vi "wfm_feature update_xygraph_x_scale.vi"(8 "error in (no error)":errorcluster, 10 "NewRange":T1, 11 "wfm_feature in":refnum<class "wfm_feature.lvclass">) -> (0 "error out":errorcluster, 3 "wfm_feature out":refnum<class "wfm_feature.lvclass">)   [LabVIEW 2018, in "wfm_feature.lvclass"]
uses:
  wfm_feature.lvclass
  <vilib>/Utility/miscctls.llb/LVRangeTypeDef.ctl
  wfm_feature.lvclass/wfm_feature.ctl
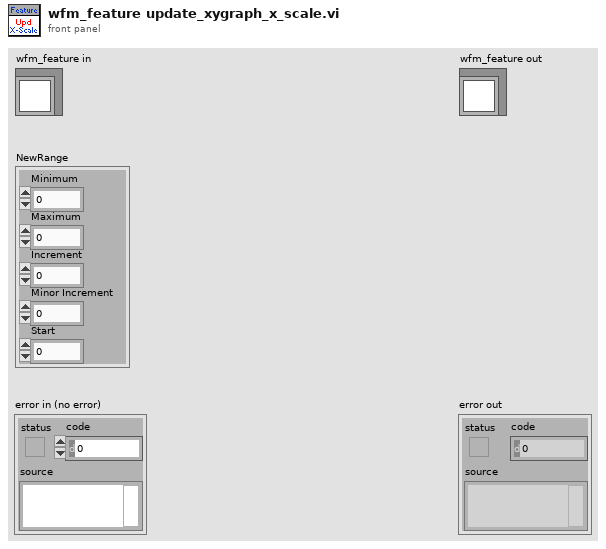
[diagram p1: front panel]
types:
  T1 = typedef "LVRangeTypeDef.ctl" = cluster{"Minimum":dbl, "Maximum":dbl, "Increment":dbl, "Minor Increment":dbl, "Start":dbl}
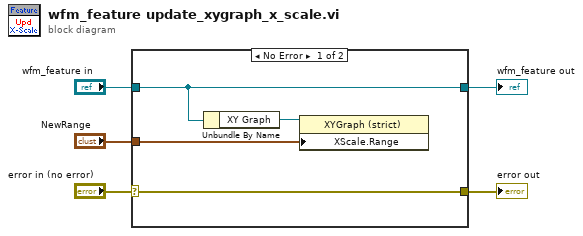
[diagram p0: block diagram]
diagram:
  n1 = case shown="No Error" "error in (no error)" {
    selector: "error in (no error)" -> [w9 w11]
    tunnel: [w9 w11] -> w4
    tunnel: [w8 w10] -> w2
    tunnel: "wfm_feature in" -> [w8 w10]
    tunnel: "NewRange" -> [w6 _]
    frame No Error {
      n2 = Unbundle By Name(w8) -> ("XY Graph"=w7:refnum<vi>)
      n3 = property class="XYGraph (strict)"(reference=w7, "XScale.Range"=w6) -> ()  [unwired: 1 in, 2 out]
    }
    frame Error {
    }
  }
  "error out" <- w4
  "wfm_feature out" <- w2
